vi "Write Lib Tokens (string).vi"(8 "error in (no error)":errorcluster, 10 "Lib Tokens":string, 11 "Lv Proj Document Type:TAF Proj Config in":refnum<class "TAF Proj Config.lvclass">) -> (0 "error out":errorcluster, 3 "Lv Proj Document Type:TAF Proj Config out":refnum<class "TAF Proj Config.lvclass">)   [LabVIEW 2021, in "TAF Proj Document Type.lvlib" / "TAF Proj Config.lvclass"]
uses:
  <vilib>/Wovalab/AntiDoc/Document Type/Add-ons/LabVIEW TAF Project/TAF Proj Config/TAF Proj Config.lvclass
  <vilib>/Wovalab/AntiDoc/Document Type/Add-ons/LabVIEW TAF Project/TAF Proj Config/TAF Proj Config.lvclass/TAF Proj Config.ctl
  <vilib>/Wovalab/AntiDoc/Utilities/Remove Empty Strings.vi
  <vilib>/AdvancedString/Split String.vi
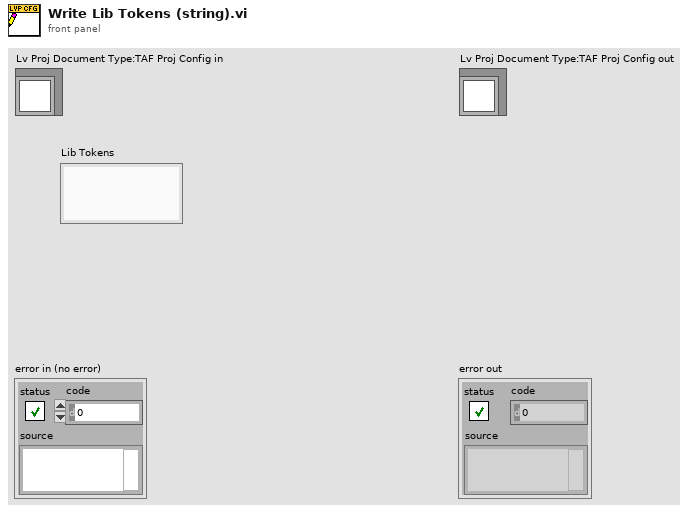
[diagram p1: front panel]
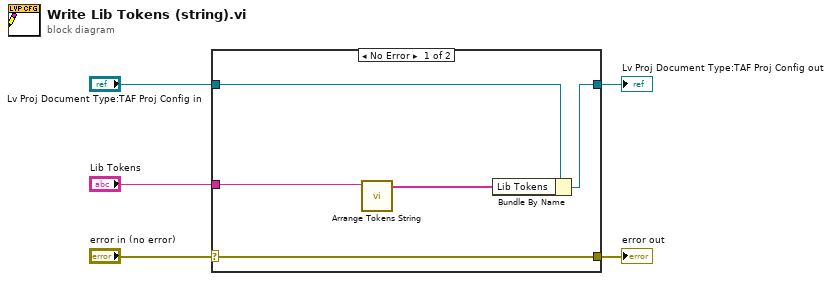
[diagram p0: block diagram]
diagram:
  n1 = case shown="No Error" "error in (no error)" {
    selector: "error in (no error)" -> [w10 w11]
    tunnel: [w10 w11] -> w4
    tunnel: [w8 w12] -> w2
    tunnel: "Lv Proj Document Type:TAF Proj Config in" -> [w9 w12]
    tunnel: "Lib Tokens" -> [w7 _]
    frame No Error {
      n2 = call <vilib>:"Arrange Tokens String.vi"("Lib Tokens"=w7) -> ("Array"=w6:string[])  [unwired: 10 in]
      n3 = Bundle By Name(cluster=w9, "Lib Tokens"=w6) -> (w8:refnum<class "TAF Proj Config.lvclass">)
    }
    frame Error {
    }
  }
  "error out" <- w4
  "Lv Proj Document Type:TAF Proj Config out" <- w2
